vi "SerialLed.vi"() -> ()   [LabVIEW 2015]
doc: "本范例根据用户指示，对串口执行读写操作。范例运行时可按下“写入”或“读取”按钮，以及修改“读数”。\n\n设置的串口参数必须匹配连接仪器或设备的参数。本范例中，“读数”参数可指定串口读取的字节数。如端口字节超过指定的字节数，超出部分将不会被读取。如端口字节数少于指定的字节数，将返回超时错误。\n\n本范例可扩展流控制选项以包括XON和XOFF，从而允许用户选择控制字符。同时，用户可启用或禁用中止符。部分设备需要通过终止符确定命令字符串的结束位置。部分设备将发送终止符以说明待读取数据的末端。本范例演示了缓冲区中检测到终止符时，结束“读取”操作或添加终止符至“写入”数据末端的方法。"
uses:
  C:/Program Files (x86)/National Instruments/LabVIEW 2015/examples/Instrument IO/Serial/support/Serial - Settings.ctl
  <vilib>/Instr/_visa.llb/VISA Configure Serial Port (Instr).vi
panel:
  in  "布尔":bool
  in  "停止":bool
  in  "VISA资源名称":refnum<visa-resource-name>="COM1"
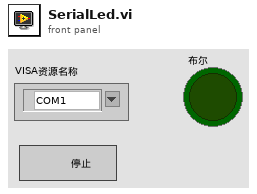
[diagram p1: front panel]
types:
  T1 = typedef "Serial - Settings.ctl" = cluster{"波特率":u32, "数据比特":u16, "奇偶":enum16{"None", "Odd", "Even", "Mark", "Space"}, "停止位":u16, "流控制":u16}
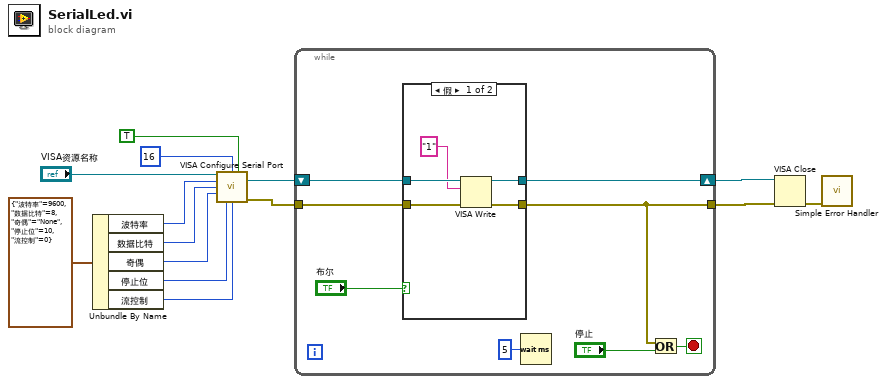
[diagram p0: block diagram]
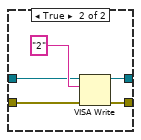
[diagram p2: hidden frame]
diagram:
  n1 = Unbundle By Name(T1 {"波特率"=9600, "数据比特"=8, "奇偶"=enum."None", "停止位"=10, "流控制"=0} ("串口设置")) -> ("波特率"=w10:u32, "数据比特"=w11:u16, "奇偶"=w12:enum16{"None", "Odd", "Even", "Mark", "Space"}, "停止位"=w13:u16, "流控制"=w4:u16)
  n2 = call-poly "VISA Configure Serial Port"("VISA resource name"="VISA资源名称", "termination char\n(0xA = '\\n' = LF)"=u8 16 ("终止符"), "Enable Termination\nChar (T)"=TRUE ("终止符时结束读取？"), "baud rate (9600)"=w10, "data bits (8)"=w11, "parity (0:none)"=w12, "stop bits (10: 1 bit)"=w13, "flow control (0:none)"=w4) -> ("VISA resource name out"=w2:refnum<visa-resource-name>, "error out"=w3:errorcluster)  [unwired: 2 in, 4 out]
  n3 = while {
    shift-right: [w16] -> w5
    shift-left: w2 -> [w22]
    tunnel: w3 -> [w21]
    tunnel: [w15] -> w6
    stop <- w19 stop-if-true
    n4 = case shown="假" "布尔" {
      tunnel: w22 -> [w27 w31]
      tunnel: w21 -> [w26 w30]
      tunnel: [w25 w29] -> w16
      tunnel: [w23 w28] -> w15
      frame False {
        n5 = VISA Write(VISA resource name=w27, write buffer="1" ("命令"), error in (no error)=w26) -> (VISA resource name out=w25:refnum<visa-resource-name>, error out=w23:errorcluster)  [unwired: 1 out]
      }
      frame True {
        n6 = VISA Write(VISA resource name=w31, write buffer="2" ("命令"), error in (no error)=w30) -> (VISA resource name out=w29:refnum<visa-resource-name>, error out=w28:errorcluster)  [unwired: 1 out]
      }
    }
    n7 = Wait (ms)(milliseconds to wait=u32 5) -> ()  [unwired: 1 out]
    n8 = Or(x=w15, y="停止") -> (x .or. y?=w19:bool)
  }
  n9 = VISA Close(VISA resource name=w5, error in (no error)=w6) -> (error out=w7:errorcluster)
  n10 = call <vilib>:"Simple Error Handler.vi"("error in (no error)"=w7) -> ()  [unwired: 1 in, 8 out]
